vi "VI Tag.vi"(6 "Is Persistent":bool, 7 "Mode":T1(ring), 8 "错误输入（无错误）":errorcluster, 9 "Value":variant, 10 "Tag Name":string, 11 "VI Ref In":refnum<vi>) -> (0 "错误输出":errorcluster, 1 "Tag Value":variant, 2 "Tag Names":string[](array[string]), 3 "VI Ref Out":refnum<vi>, 4 "Is Persistent?":bool, 5 "Succeed?":bool)   [LabVIEW 2012, in "VIRef.lvlib"]
uses:
  VIRef.lvlib
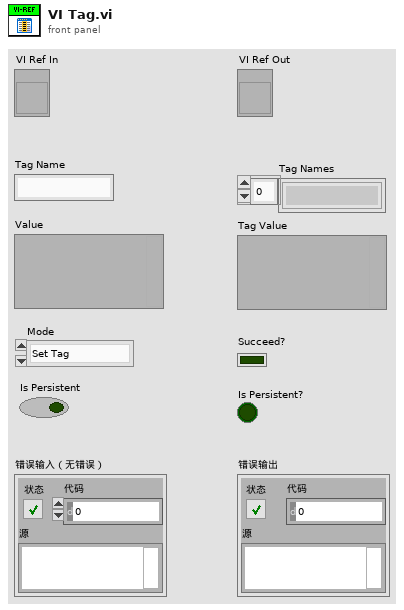
[diagram p1: front panel]
types:
  T1 = enum16{"Set Tag", "Remove Tag", "Get Tag", "Remove All Tags", "Get Tag Names"}
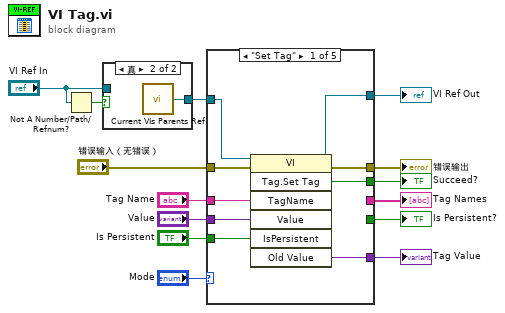
[diagram p0: block diagram]
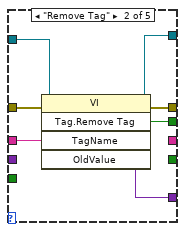
[diagram p2: hidden frame]
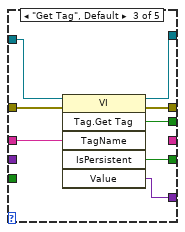
[diagram p3: hidden frame]
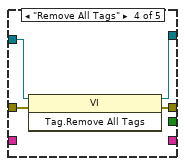
[diagram p4: hidden frame]
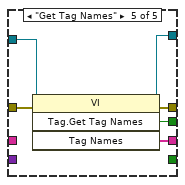
[diagram p5: hidden frame]
diagram:
  n1 = Not A Number/Path/Refnum?(number/path/refnum="VI Ref In") -> (NaN/Path/Refnum?=w13:bool)
  n2 = case shown="真" w13 {
    tunnel: [w15 w16] -> w4
    tunnel: "VI Ref In" -> [w15 _]
    frame False {
    }
    frame True {
      n3 = call "Current VIs Parents Ref.vi"() -> ("Calling VI's Reference"=w16:refnum<vi>)  [unwired: 2 in]
    }
  }
  n4 = case shown="\"Set Tag\"" "Mode" {
    tunnel: [w25 w28 w35 _ _] -> w11
    tunnel: "Is Persistent" -> [w24 _ _ _ _]
    tunnel: "Tag Name" -> [w23 w29 w33 _ _]
    tunnel: "Value" -> [w22 _ _ _ _]
    tunnel: "错误输入（无错误）" -> [w21 w32 w40 w43 w49]
    tunnel: [w20 w27 w37 w42 w47] -> w6
    tunnel: [w19 w26 w36 _ w45] -> w5
    tunnel: w4 -> [w18 w31 w39 w44 w50]
    tunnel: [_ _ w34 _ _] -> w3
    tunnel: [w17 w30 w38 w41 w48] -> w2
    tunnel: [_ _ _ _ w46] -> w1
    frame "Set Tag" {
      n5 = invoke class="VI" method="Tag.Set Tag"(reference=w18, error in=w21, "TagName"=w23, "Value"=w22, "IsPersistent"=w24) -> (reference out=w17:refnum<vi>, error out=w20:errorcluster, "SetTag"=w19:bool, "Old Value"=w25:variant)  [unwired: 2 in, 3 out]
    }
    frame "Remove Tag" {
      n6 = invoke class="VI" method="Tag.Remove Tag"(reference=w31, error in=w32, "TagName"=w29) -> (reference out=w30:refnum<vi>, error out=w27:errorcluster, "RemoveTag"=w26:bool, "OldValue"=w28:variant)  [unwired: 2 in, 1 out]
    }
    frame "Get Tag", Default {
      n7 = invoke class="VI" method="Tag.Get Tag"(reference=w39, error in=w40, "TagName"=w33) -> (reference out=w38:refnum<vi>, error out=w37:errorcluster, "GetTag"=w36:bool, "IsPersistent"=w34:bool, "Value"=w35:variant)  [unwired: 3 in, 1 out]
    }
    frame "Remove All Tags" {
      n8 = invoke class="VI" method="Tag.Remove All Tags"(reference=w44, error in=w43) -> (reference out=w41:refnum<vi>, error out=w42:errorcluster)  [unwired: 1 in, 1 out]
    }
    frame "Get Tag Names" {
      n9 = invoke class="VI" method="Tag.Get Tag Names"(reference=w50, error in=w49) -> (reference out=w48:refnum<vi>, error out=w47:errorcluster, "Tag.Get Tag Names"=w45:bool, "Tag Names"=w46:string[])  [unwired: 2 in]
    }
  }
  "VI Ref Out" <- w2
  "Succeed?" <- w5
  "Tag Value" <- w11
  "错误输出" <- w6
  "Is Persistent?" <- w3
  "Tag Names" <- w1
